vi "OutProc.vi"(7 "Motor Cluster In":cluster{T1[], T10[]}, 11 "ActuatorInputs":T12) -> (3 "ActuatorInputsOut":T12)   [LabVIEW 2014]
uses:
  Typedefs/ActuatorInputs.ctl
  <vilib>/Rock Robotics/WPI/MotorControl/WPI_MotorControlDeviceRef.ctl
  <vilib>/Rock Robotics/WPI/MotorControl/WPI_MotorControlType.ctl
  <vilib>/Rock Robotics/SystemInterfaces/Typedef/FPGA_TypedefDigitalModule.ctl
  <vilib>/Rock Robotics/SystemInterfaces/DIO/FPGA_DIOPWMChannel.ctl
  <vilib>/Rock Robotics/WPI/PWM/WPI_PWMDeadband.ctl
  <vilib>/Rock Robotics/WPI/CAN/Jaguar/SubVIs/WPI_CANJaguar_ControlMode.ctl
  <vilib>/Rock Robotics/WPI/CAN/TalonSRX/WPI_CANTalonSRX_APIControlMode.ctl
  <vilib>/Rock Robotics/WPI/PWM/WPI_PWMTransform_ConPane.ctl
  <vilib>/Rock Robotics/WPI/Solenoid/WPI_SolenoidDevRef.ctl
  <vilib>/Rock Robotics/WPI/Solenoid/WPI_SolenoidChannel.ctl
  <vilib>/Rock Robotics/WPI/Solenoid/Deprecated/WPI_SolenoidSetBool.vi
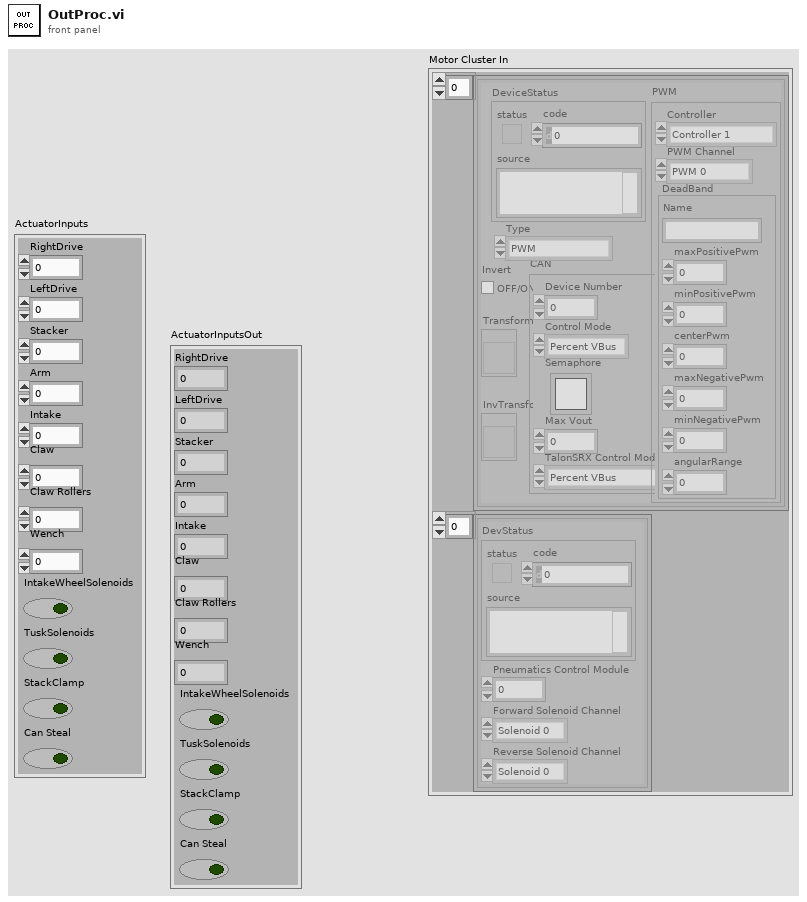
[diagram p1: front panel]
types:
  T1 = typedef "WPI_MotorControlDeviceRef.ctl" = cluster{"DeviceStatus":errorcluster, "Type":T2, "PWM":cluster{"Controller":T3, "PWM Channel":T4, "DeadBand":T5}, "CAN":cluster{"Device Number":u8, "Control Mode":T6, "Semaphore":T7, "Max Vout":dbl, "TalonSRX Control Mode":T8}, "Invert":bool, "TransformRef":T9, "InvTransformRef":T9}
  T2 = typedef "WPI_MotorControlType.ctl" = enum16{"PWM", "CAN", "CANTalonSRX"}
  T3 = typedef "FPGA_TypedefDigitalModule.ctl" = enum16{"Controller 1"}
  T4 = typedef "FPGA_DIOPWMChannel.ctl" = enum8{"PWM 0", "PWM 1", "PWM 2", "PWM 3", "PWM 4", "PWM 5", "PWM 6", "PWM 7", "PWM 8", "PWM 9", "PWM MXP 0", "PWM MXP 1", "PWM MXP 2", "PWM MXP 3", "PWM MXP 4", "PWM MXP 5", "PWM MXP 6", "PWM MXP 7", "PWM MXP 8", "PWM MXP 9", "Invalid"}
  T5 = typedef "WPI_PWMDeadband.ctl" = cluster{"Name":string, "maxPositivePwm":i32, "minPositivePwm":i32, "centerPwm":i32, "maxNegativePwm":i32, "minNegativePwm":i32, "angularRange":u16}
  T6 = typedef "WPI_CANJaguar_ControlMode.ctl" = enum8{"Percent VBus", "Current", "Speed", "Position", "Voltage"}
  T7 = typedef "Semaphore RefNum" = refnum<k1>
  T8 = typedef "WPI_CANTalonSRX_APIControlMode.ctl" = enum8{"Percent VBus", "Speed", "Position", "Slave", "Unchanged / Invalid"}
  T9 = typedef "WPI_PWMTransform_ConPane.ctl" = refnum<vi>
  T10 = typedef "WPI_SolenoidDevRef.ctl" = cluster{"DevStatus":errorcluster, "Pneumatics Control Module":u8, "Forward Solenoid Channel":T11, "Reverse Solenoid Channel":T11}
  T11 = typedef "WPI_SolenoidChannel.ctl" = enum8{"Solenoid 0", "Solenoid 1", "Solenoid 2", "Solenoid 3", "Solenoid 4", "Solenoid 5", "Solenoid 6", "Solenoid 7", "Invalid"}
  T12 = typedef "ActuatorInputs.ctl" = cluster{"RightDrive":dbl, "LeftDrive":dbl, "Stacker":dbl, "Arm":dbl, "Intake":sgl, "Claw":dbl, "Claw Rollers":i8, "Wench":dbl, "IntakeWheelSolenoids":bool, "TuskSolenoids":bool, "StackClamp":bool, "Can Steal":bool}
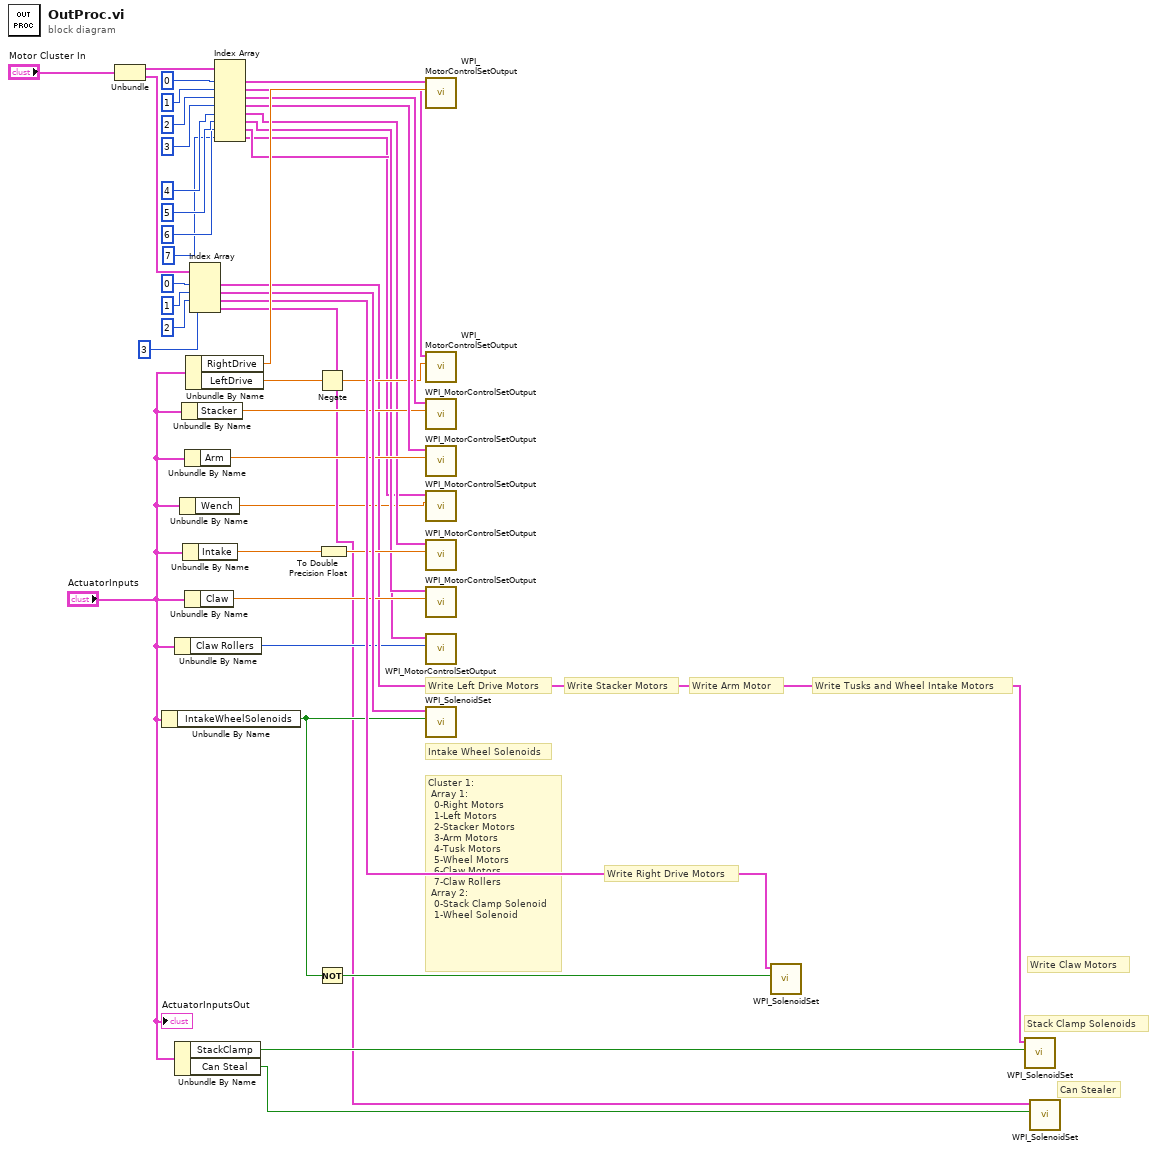
[diagram p0: block diagram]
diagram:
  # "Can Stealer"
  # "Intake Wheel Solenoids"
  # "Stack Clamp Solenoids"
  # "Write Claw Motors"
  # "Write Tusks and Wheel Intake Motors"
  # "Write Arm Motor"
  # "Write Stacker Motors"
  # "Cluster 1:\n Array 1:\n  0-Right Motors\n  1-Left Motors\n  2-Stacker Motors\n  3-Arm Motors\n  4-Tusk Motors\n  5-Wheel Motors\n  6-Claw Motors\n  7-Claw Rollers\n Array 2:\n  0-Stack Clamp Solenoid\n  1-Wheel Solenoid"
  # "Write Left Drive Motors"
  # "Write Right Drive Motors"
  n1 = Unbundle("Motor Cluster In") -> (w32:T1[], w30:T10[])
  n2 = Unbundle By Name("ActuatorInputs") -> ("IntakeWheelSolenoids"=w18:bool)
  n3 = Unbundle By Name("ActuatorInputs") -> ("Claw Rollers"=w14:i8)
  n4 = Unbundle By Name("ActuatorInputs") -> ("StackClamp"=w16:bool, "Can Steal"=w6:bool)
  n5 = Unbundle By Name("ActuatorInputs") -> ("Wench"=w3:dbl)
  n6 = Unbundle By Name("ActuatorInputs") -> ("Stacker"=w22:dbl)
  n7 = Unbundle By Name("ActuatorInputs") -> ("Intake"=w31:sgl)
  n8 = Unbundle By Name("ActuatorInputs") -> ("Arm"=w21:dbl)
  n9 = Unbundle By Name("ActuatorInputs") -> ("Claw"=w23:dbl)
  n10 = Unbundle By Name("ActuatorInputs") -> ("RightDrive"=w42:dbl, "LeftDrive"=w29:dbl)
  n11 = Index Array(array=w30, index #1=0 ("index"), index #2=1 ("index"), index #3=2 ("index"), index #4=3 ("index")) -> (element #1=w15:T10, element #2=w26:T10, element #3=w24:T10, element #4=w5:T10)
  n12 = Index Array(array=w32, index #1=0 ("index"), index #2=1 ("index"), index #3=2 ("index"), index #4=3 ("index"), index #5=4 ("index"), index #6=5 ("index"), index #7=6 ("index"), index #8=7 ("index")) -> (element #1=w40:T1, element #2=w38:T1, element #3=w35:T1, element #4=w34:T1, element #5=w13:T1, element #6=w11:T1, element #7=w8:T1, element #8=w1:T1)
  n13 = Negate(x=w29) -> (-x=w19:dbl)
  n14 = Not(x=w18) -> (.not. x?=w17:bool)
  n15 = To Double Precision Float(number=w31) -> (double precision float=w20:dbl)
  n16 = call <vilib>:"WPI_MotorControlSetOutput.vi"("Output"=w42, "MotorControlDevRef"=w40) -> ()  [unwired: 7 in, 3 out]
  n17 = call <vilib>:"WPI_MotorControlSetOutput.vi"("Output"=w19, "MotorControlDevRef"=w38) -> ()  [unwired: 7 in, 3 out]
  n18 = call <vilib>:"WPI_MotorControlSetOutput.vi"("Output"=w22, "MotorControlDevRef"=w35) -> ()  [unwired: 7 in, 3 out]
  n19 = call <vilib>:"WPI_MotorControlSetOutput.vi"("Output"=w21, "MotorControlDevRef"=w34) -> ()  [unwired: 7 in, 3 out]
  n20 = call <vilib>:"WPI_MotorControlSetOutput.vi"("Output"=w3, "MotorControlDevRef"=w1) -> ()  [unwired: 7 in, 3 out]
  n21 = call <vilib>:"WPI_MotorControlSetOutput.vi"("Output"=w20, "MotorControlDevRef"=w13) -> ()  [unwired: 7 in, 3 out]
  n22 = call <vilib>:"WPI_MotorControlSetOutput.vi"("Output"=w23, "MotorControlDevRef"=w11) -> ()  [unwired: 7 in, 3 out]
  n23 = call <vilib>:"WPI_MotorControlSetOutput.vi"("Output"=w14, "MotorControlDevRef"=w8) -> ()  [unwired: 7 in, 3 out]
  n24 = call-poly <vilib>:"WPI_SolenoidSet.vi"("Value"=w18, "SolenoidDevRef"=w26) -> ()  [unwired: 8 in, 2 out]
  n25 = call-poly <vilib>:"WPI_SolenoidSet.vi"("Value"=w17, "SolenoidDevRef"=w24) -> ()  [unwired: 8 in, 2 out]
  n26 = call-poly <vilib>:"WPI_SolenoidSet.vi"("Value"=w16, "SolenoidDevRef"=w15) -> ()  [unwired: 8 in, 2 out]
  n27 = call-poly <vilib>:"WPI_SolenoidSet.vi"("Value"=w6, "SolenoidDevRef"=w5) -> ()  [unwired: 8 in, 2 out]
  "ActuatorInputsOut" <- "ActuatorInputs"
